vi "Initialization phase.vi"(8 "error in (no error)":errorcluster, 11 "Programming Logic in":refnum<class "Programming Logic.lvclass">) -> (0 "error out":errorcluster, 3 "Programming Logic out":refnum<class "Programming Logic.lvclass">)   [LabVIEW 2014, in "Files Library.lvlib" / "Programming Logic.lvclass"]
uses:
  Programming Logic.lvclass
  Programming Logic.lvclass/Programming Logic.ctl
  <vilib>/NI/Modbus Library/API/Wrapper/Create Serial Master.vi
  <vilib>/NI/Modbus Library/API/Wrapper/API Main.lvlib
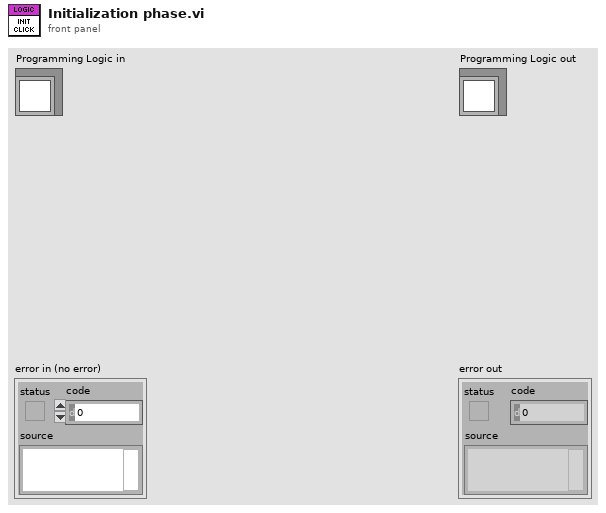
[diagram p1: front panel]
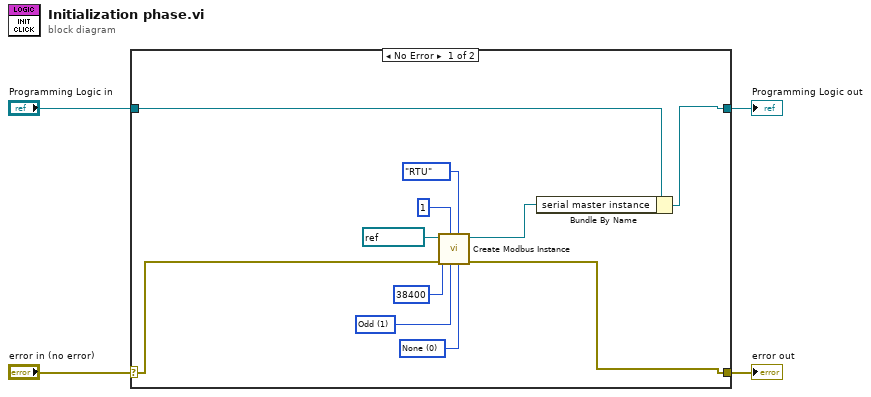
[diagram p0: block diagram]
diagram:
  n1 = case shown="No Error" "error in (no error)" {
    selector: "error in (no error)" -> [w8 w17]
    tunnel: [w7 w17] -> w3
    tunnel: [w9 w16] -> w1
    tunnel: "Programming Logic in" -> [w6 w16]
    frame No Error {
      w13 = u16 0 items=["None", "XON/XOFF", "RTS/CTS", "XON/XOFF & RTS/CTS", "DTR/DSR", "XON/XOFF & DTR/DSR"] ("flow control (none)")
      w14 = u16 1 items=["None", "Odd", "Even", "Mark", "Space"] ("parity (even)")
      n2 = call-poly <vilib>:"Create Modbus Instance.vi"("flow control (none)"=w13, "serial type"=enum16{"RTU", "ASCII"}."RTU", "parity (even)"=w14, "unit ID"=u8 1, "error in"=w8, "baud rate"=u32 38400, "VISA resource name"=refnum<visa-resource-name> "COM1") -> ("error out"=w7:errorcluster, "serial master instance"=w10:refnum<class "Modbus Master.lvclass">)  [unwired: 3 in]
      n3 = Bundle By Name(cluster=w6, "serial master instance"=w10) -> (w9:refnum<class "Programming Logic.lvclass">)
    }
    frame Error {
    }
  }
  "error out" <- w3
  "Programming Logic out" <- w1
